vi "Delete Message (Batch).vi"(8 "error in (no error)":errorcluster, 10 "Receipt Handles":string[](array[string]), 11 "SQS in":refnum<class "Queue.lvclass">) -> (0 "error out":errorcluster, 3 "SQS out":refnum<class "Queue.lvclass">)   [LabVIEW 2015, in "NI_AWS_SQS.lvlib" / "Queue.lvclass"]
uses:
  Queue.lvclass
  Core/HTTP Request/Name Value Pair.ctl
  Core/HTTP Request/Request Options.ctl
  Queue.lvclass/Queue.ctl
  Read Account Number.vi
  Read Name.vi
  Core/HTTP Request/HTTP Request.lvclass
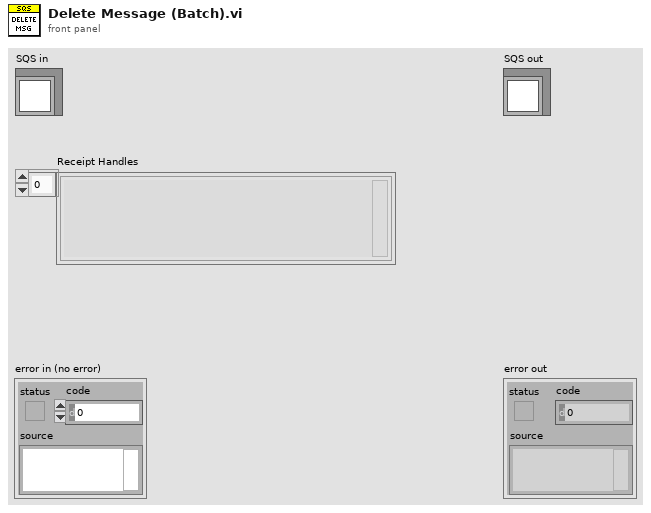
[diagram p1: front panel]
types:
  T1 = typedef "NI_AWS_Core.lvlib/HTTP Request.lvclass/Request Options.ctl" = cluster{"request headers":T2[], "request parameters":T2[], "request body":string}
  T2 = typedef "NI_AWS_Core.lvlib/HTTP Request.lvclass/Name Value Pair.ctl" = cluster{"name":string, "value":string}
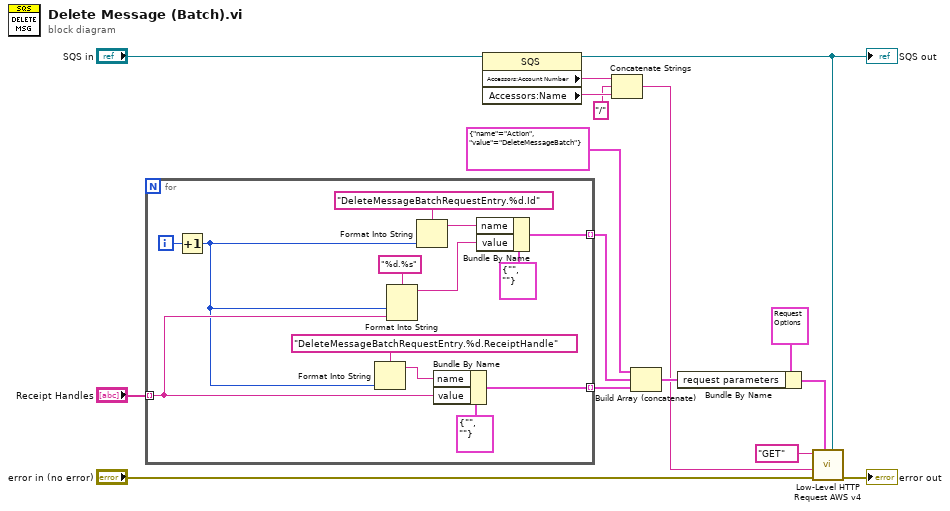
[diagram p0: block diagram]
diagram:
  n1 = for {
    tunnel: [w28] -> w4 mode=indexing
    tunnel: "Receipt Handles" -> [w18] mode=indexing
    tunnel: [w25] -> w1 mode=indexing
    i -> [w26]
    n2 = Increment(x=w26) -> (x+1=w17:i32)
    n3 = Format Into String(format string="DeleteMessageBatchRequestEntry.%d.ReceiptHandle" ("name"), w17) -> (resulting string=w19:string)  [unwired: 2 in, 1 out]
    n4 = Format Into String(format string="%d.%s", w17, w18) -> (resulting string=w21:string)  [unwired: 2 in, 1 out]
    n5 = Format Into String(format string="DeleteMessageBatchRequestEntry.%d.Id" ("name"), w17) -> (resulting string=w24:string)  [unwired: 2 in, 1 out]
    n6 = Bundle By Name(cluster=T2 {"name"="", "value"=""} ("element"), "name"=w19, "value"=w18) -> (w28:T2)
    n7 = Bundle By Name(cluster=T2 {"name"="", "value"=""} ("element"), "name"=w24, "value"=w21) -> (w25:T2)
  }
  n8 = property class="SQS"(reference="SQS in") -> (reference out=w9:refnum<class "Queue.lvclass">, "Accessors:Account Number"=w8:string, "Accessors:Name"=w7:string)  [unwired: 1 in, 1 out]
  "SQS out" <- w9
  n9 = Concatenate Strings(w8, "/", w7) -> (w5:string)
  n10 = Build Array (concatenate)(T2 {"name"="Action", "value"="DeleteMessageBatch"} ("Cluster"), w1, w4) -> (w10:T2[])
  n11 = Bundle By Name(cluster=T1 {"request headers"=[], "request parameters"=[{"name"="Action", "value"="ListQueues"}], "request body"=""} ("Request Options"), "request parameters"=w10) -> (w11:T1)
  n12 = call "Low-Level HTTP Request AWS v4.vi"("AWS Core"=w9, "Request Options"=w11, "error in (no error)"="error in (no error)", "URL Suffix"=w5, "HTTP-Verb"="GET") -> ("error out"=→"error out":errorcluster)  [unwired: 4 in, 2 out]
